vi "SMTP Email Convert To JIS.vi"(10 "character set":string, 11 "text in":string) -> (3 "text out":string)   [LabVIEW 2012, in "NewNI_SMTPEmail.lvlib"]
doc: "This VI converts the input code to JIS (ISO-2022-JP)."
uses:
  NewNI_SMTPEmail.lvlib
panel:
  out "character set out":string
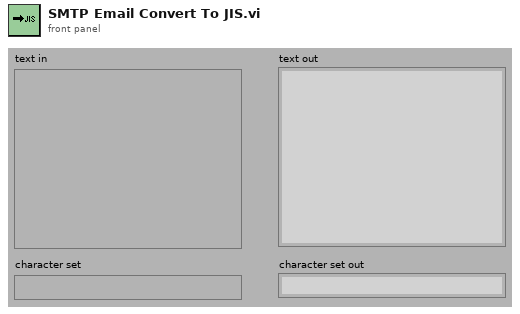
[diagram p1: front panel]
types:
  T1 = enum16{"NOTSET", "NEW", "OLD", "NEC", "EUC", "SJIS", "EUCORSJIS", "ASCII"}
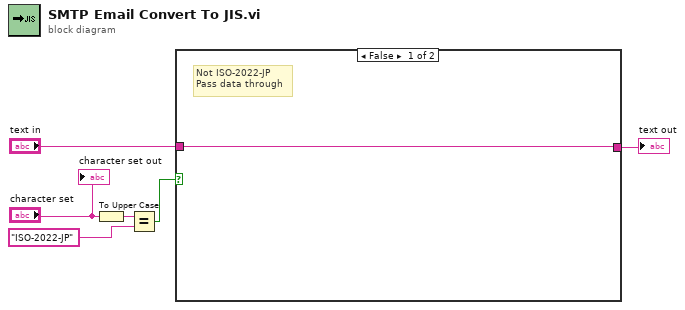
[diagram p0: block diagram]
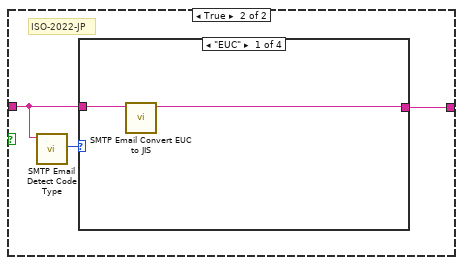
[diagram p2: hidden frame]
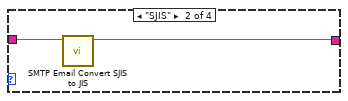
[diagram p3: hidden frame]
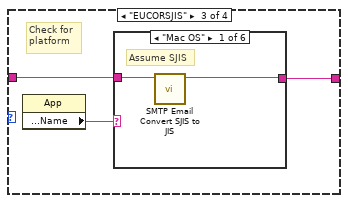
[diagram p4: hidden frame]
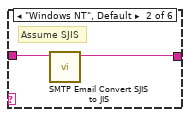
[diagram p5: hidden frame]
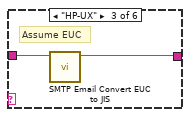
[diagram p6: hidden frame]
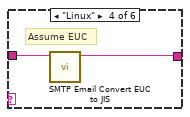
[diagram p7: hidden frame]
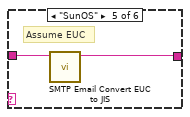
[diagram p8: hidden frame]
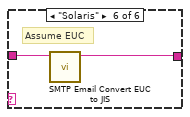
[diagram p9: hidden frame]
diagram:
  n1 = To Upper Case(1:"character set") -> (0:w5:string)
  n2 = Equal?(x=w5, y="ISO-2022-JP") -> (x = y?=w2:bool)
  n3 = case shown="False" w2 {
    tunnel: "text in" -> [w7 w9]
    tunnel: [w7 w8] -> w1
    frame False {
      # "Not ISO-2022-JP\nPass data through"
    }
    frame True {
      # "ISO-2022-JP"
      n4 = call "SMTP Email Detect Code Type.vi"("text in"=w9) -> ("code type"=w10:T1)  [unwired: 10 out]
      n5 = case shown="\"EUC\"" w10 {
        tunnel: w9 -> [w12 w14 w16 w30]
        tunnel: [w11 w13 w15 w30] -> w8
        frame "EUC" {
          n6 = call "SMTP Email Convert EUC to JIS.vi"("text in"=w12) -> ("text out"=w11:string)  [unwired: 10 out]
        }
        frame "SJIS" {
          n7 = call "SMTP Email Convert SJIS to JIS.vi"("text in"=w14) -> ("text out"=w13:string)  [unwired: 1 in, 9 out]
        }
        frame "EUCORSJIS" {
          # "Check for\nplatform"
          n8 = property class="App"() -> ("Operating System:Name"=w17:string)  [unwired: 2 in, 2 out]
          n9 = case shown="\"Mac OS\"" w17 {
            tunnel: w16 -> [w19 w21 w23 w25 w27 w29]
            tunnel: [w18 w20 w22 w24 w26 w28] -> w15
            frame "Mac OS" {
              # "Assume SJIS"
              n10 = call "SMTP Email Convert SJIS to JIS.vi"("text in"=w19) -> ("text out"=w18:string)  [unwired: 1 in, 9 out]
            }
            frame "Windows NT", Default {
              # "Assume SJIS"
              n11 = call "SMTP Email Convert SJIS to JIS.vi"("text in"=w21) -> ("text out"=w20:string)  [unwired: 1 in, 9 out]
            }
            frame "HP-UX" {
              # "Assume EUC"
              n12 = call "SMTP Email Convert EUC to JIS.vi"("text in"=w23) -> ("text out"=w22:string)  [unwired: 10 out]
            }
            frame "Linux" {
              # "Assume EUC"
              n13 = call "SMTP Email Convert EUC to JIS.vi"("text in"=w25) -> ("text out"=w24:string)  [unwired: 10 out]
            }
            frame "SunOS" {
              # "Assume EUC"
              n14 = call "SMTP Email Convert EUC to JIS.vi"("text in"=w27) -> ("text out"=w26:string)  [unwired: 10 out]
            }
            frame "Solaris" {
              # "Assume EUC"
              n15 = call "SMTP Email Convert EUC to JIS.vi"("text in"=w29) -> ("text out"=w28:string)  [unwired: 10 out]
            }
          }
        }
        frame "ASCII", Default {
          # "If code type is not of type\nSJIS or EUC, then do nothing"
        }
      }
    }
  }
  "text out" <- w1
  "character set out" <- "character set"
